vi "getXMLTestCases.vi"(9 "indent level":i32, 10 "testcases":T1[](array[typedef])) -> (2 "XML testcases":string[](array[string]))   [LabVIEW 2013, in "Caraya.lvlib" / "Test Report.JUnit.lvclass"]
uses:
  Test Report.JUnit.lvclass
  testcase -- cluster.ctl
  Test Report/Test Report.lvclass
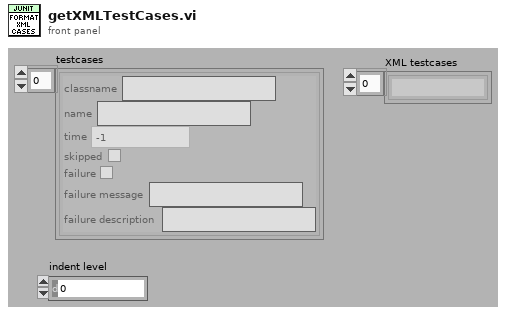
[diagram p1: front panel]
types:
  T1 = typedef "Caraya.lvlib/Test Report.JUnit.lvclass/testcase -- cluster.ctl" = cluster{"classname":string, "name":string, "time":dbl, "skipped":bool, "failure":bool, "failure message":string, "failure description":string}
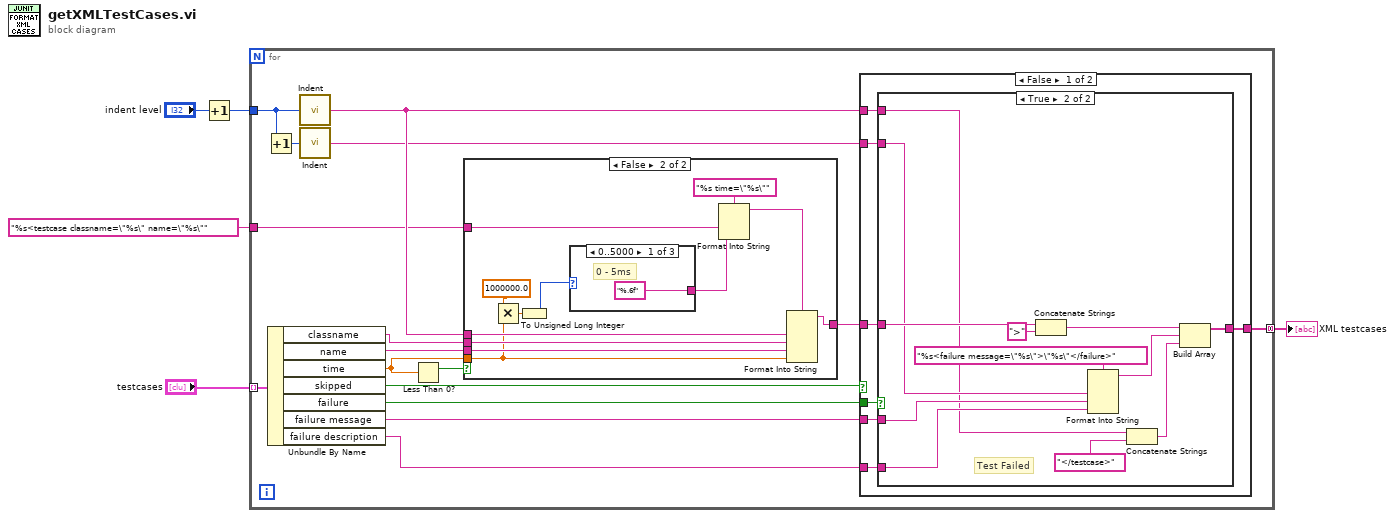
[diagram p0: block diagram]
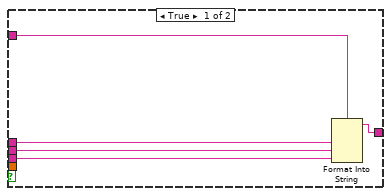
[diagram p2: hidden frame]
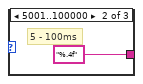
[diagram p3: hidden frame]
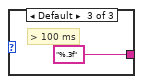
[diagram p4: hidden frame]
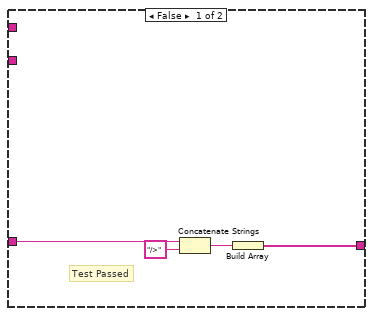
[diagram p5: hidden frame]
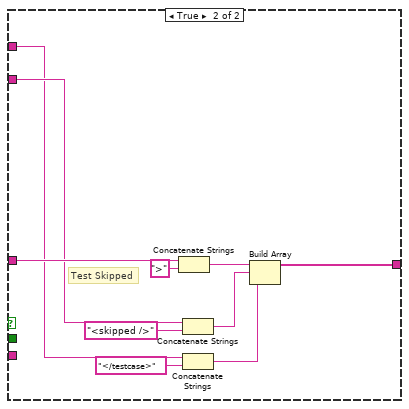
[diagram p6: hidden frame]
diagram:
  n1 = Increment(x="indent level") -> (x+1=w3:i32)
  n2 = for {
    tunnel: "testcases" -> [w21] mode=indexing
    tunnel: w3 -> [w13]
    tunnel: [w9] -> w2 mode=concatenating
    tunnel: "%s<testcase classname=\"%s\" name=\"%s\"" -> [w6]
    n3 = Increment(x=w13) -> (x+1=w11:i32)
    n4 = Unbundle By Name(w21) -> ("classname"=w19:string, "name"=w20:string, "time"=w8:dbl, "skipped"=w18:bool, "failure"=w17:bool, "failure message"=w16:string, "failure description"=w15:string)
    n5 = call "Indent.vi"("Numeric"=w13) -> ("string"=w12:string)
    n6 = call "Indent.vi"("Numeric"=w11) -> ("string"=w10:string)
    n7 = Less Than 0?(x=w8) -> (x < 0?=w7:bool)
    n8 = case shown="False" w7 {
      tunnel: w20 -> [w26 w38]
      tunnel: w19 -> [w25 w37]
      tunnel: [w24 w36] -> w14
      tunnel: w12 -> [w23 w35]
      tunnel: w8 -> [_ w29]
      tunnel: w6 -> [w22 w34]
      frame True {
        n9 = Format Into String(format string=w22, w23, w25, w26) -> (resulting string=w24:string)  [unwired: 2 in, 1 out]
      }
      frame False {
        n10 = Multiply(x=1000000.0 ("y"), y=w29) -> (x*y=w31:dbl)
        n11 = To Unsigned Long Integer(number=w31) -> (unsigned 32bit integer=w28:u32)
        n12 = case shown="0..5000" w28 {
          tunnel: ["%.6f" "%.4f" "%.3f"] -> w27
          frame 0..5000 {
            # "0 - 5ms"
          }
          frame 5001..100000 {
            # "5 - 100ms"
          }
          frame Default {
            # "> 100 ms"
          }
        }
        n13 = Format Into String(format string="%s time=\"%s\"", w34, w27) -> (resulting string=w32:string)  [unwired: 2 in, 1 out]
        n14 = Format Into String(format string=w32, w35, w37, w38, w29) -> (resulting string=w36:string)  [unwired: 2 in, 1 out]
      }
    }
    n15 = case shown="False" w18 {
      tunnel: [w47 w74] -> w9
      tunnel: w17 -> [w48 _]
      tunnel: w16 -> [w46 _]
      tunnel: w15 -> [w45 _]
      tunnel: w14 -> [w44 w72]
      tunnel: w10 -> [w43 w66]
      tunnel: w12 -> [w42 w65]
      frame False {
        n16 = case shown="True" w48 {
          tunnel: [w49 w57] -> w47
          tunnel: w46 -> [_ w62]
          tunnel: w45 -> [_ w61]
          tunnel: w44 -> [w51 w60]
          tunnel: w43 -> [_ w56]
          tunnel: w42 -> [_ w55]
          frame False {
            # "Test Passed"
            n17 = Concatenate Strings(w51, "/>" ("string")) -> (w50:string)
            n18 = Build Array(w50) -> (w49:string[])
          }
          frame True {
            # "Test Failed"
            n19 = Concatenate Strings(w60, ">" ("string")) -> (w58:string)
            n20 = Format Into String(format string="%s<failure message=\"%s\">\"%s\"</failure>", w56, w62, w61) -> (resulting string=w64:string)  [unwired: 2 in, 1 out]
            n21 = Concatenate Strings(w55, "</testcase>") -> (w53:string)
            n22 = Build Array(w58, w64, w53) -> (w57:string[])
          }
        }
      }
      frame True {
        # "Test Skipped"
        n23 = Concatenate Strings(w72, ">" ("string")) -> (w71:string)
        n24 = Concatenate Strings(w66, "<skipped />") -> (w67:string)
        n25 = Concatenate Strings(w65, "</testcase>") -> (w69:string)
        n26 = Build Array(w71, w67, w69) -> (w74:string[])
      }
    }
  }
  "XML testcases" <- w2
